vi "NicmosOpen.vi"(0 "FilterList":T1, 2 "MASKBANKS":T3, 3 "NICMOS Port":refnum<visa-resource-name>="COM1", 9 "error in (no error)":errorcluster caption="entrée d'erreur") -> (1 "NICMOS task out":refnum<k21>, 6 "error out":errorcluster caption="sortie d'erreur")   [LabVIEW 2009]
doc: "Ouverture des communications avec l'électronique, passage en mode déclanché et écriture des masques si besoin."
uses:
  Controls/NICMOS.MASKBANKS.ctl
  Controls/NICMOS.FILTERLIST.ctl
  Controls/NICMOS.FILTER.ctl
  NicmosGlobal.vi
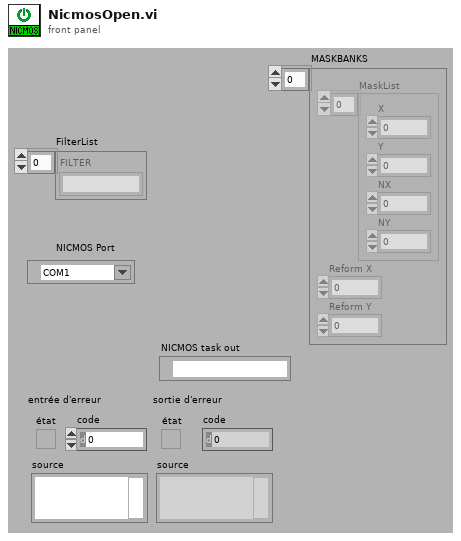
[diagram p1: front panel]
types:
  T1 = typedef "NICMOS.FILTERLIST.ctl" = T2[]
  T2 = typedef "NICMOS.FILTER.ctl" = string
  T3 = typedef "NICMOS.MASKBANKS.ctl" = cluster{"MaskList":cluster{"X":i32, "Y":i32, "NX":i32, "NY":i32}[], "Reform X":i32, "Reform Y":i32}[]
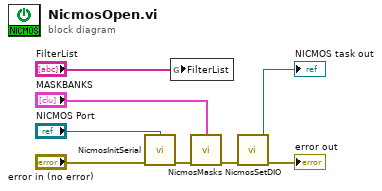
[diagram p0: block diagram]
diagram:
  n1 = call "NicmosInitSerial.vi"("error in (no error)"="error in (no error)", "Port Nicmos"="NICMOS Port") -> ("error out"=w7:errorcluster)  [unwired: 3 in]
  n2 = global write "NicmosGlobal.vi" "FilterList"("FilterList") -> ()
  n3 = call "NicmosMasks.vi"("MASKBANKS"="MASKBANKS", "Error in (no error)"=w7) -> ("Error out"=w5:errorcluster)  [unwired: 7 in]
  n4 = call "NicmosSetDIO.vi"("error in (no error)"=w5) -> ("NICMOS task out"=→"NICMOS task out":refnum<k21>, "error out"=→"error out":errorcluster)  [unwired: 7 in]
